vi "FPGA(test).vi"() -> ()   [LabVIEW 2019]
uses:
  <vilib>/rvi/Emulation/niFpgaGetClockAttributes.vi
  <vilib>/rvi/Emulation/niFpgaSctlEmulationGetInTimedLoop.vi
  <vilib>/rvi/Emulation/niFpgaEmulationReportErrorSimple.vi
  <vilib>/rvi/Emulation/niFpgaProcessEmulError.vi
  <vilib>/rvi/eio/common/nirviEmuTemplateMethod_errors.vi
  <vilib>/rvi/Emulation/niFpgaCriticalErrorInLSC.vi
  <vilib>/eio/EIONode/EIONode.xnode
panel:
  in  "pwm input(escon)":i32
  in  "Enable (escon)":bool
  in  "T(escon)":i32=20000
  out "Encoder(escon)":i32
  out "Encoder  (4x)":i32
  out "Encoder  (1x)":i32
  in  "encoder reset":bool
  in  "Enable":bool
  out "Encoder  (2x)":i32
  in  "stop":bool
  in  "T":i32=800000
  in  "pwm input":i32
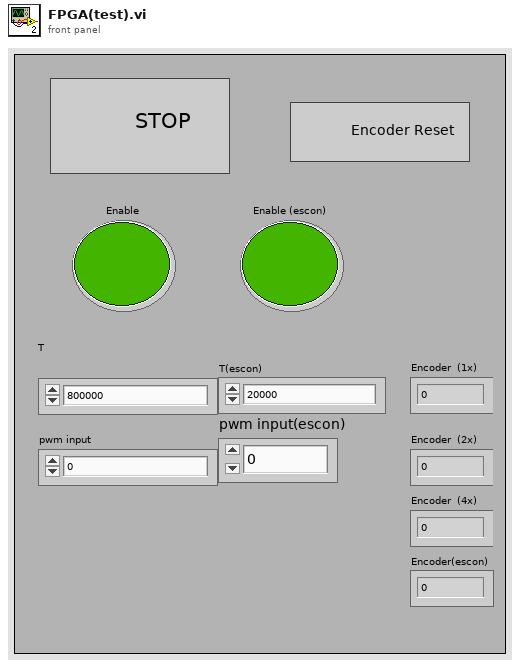
[diagram p1: front panel]
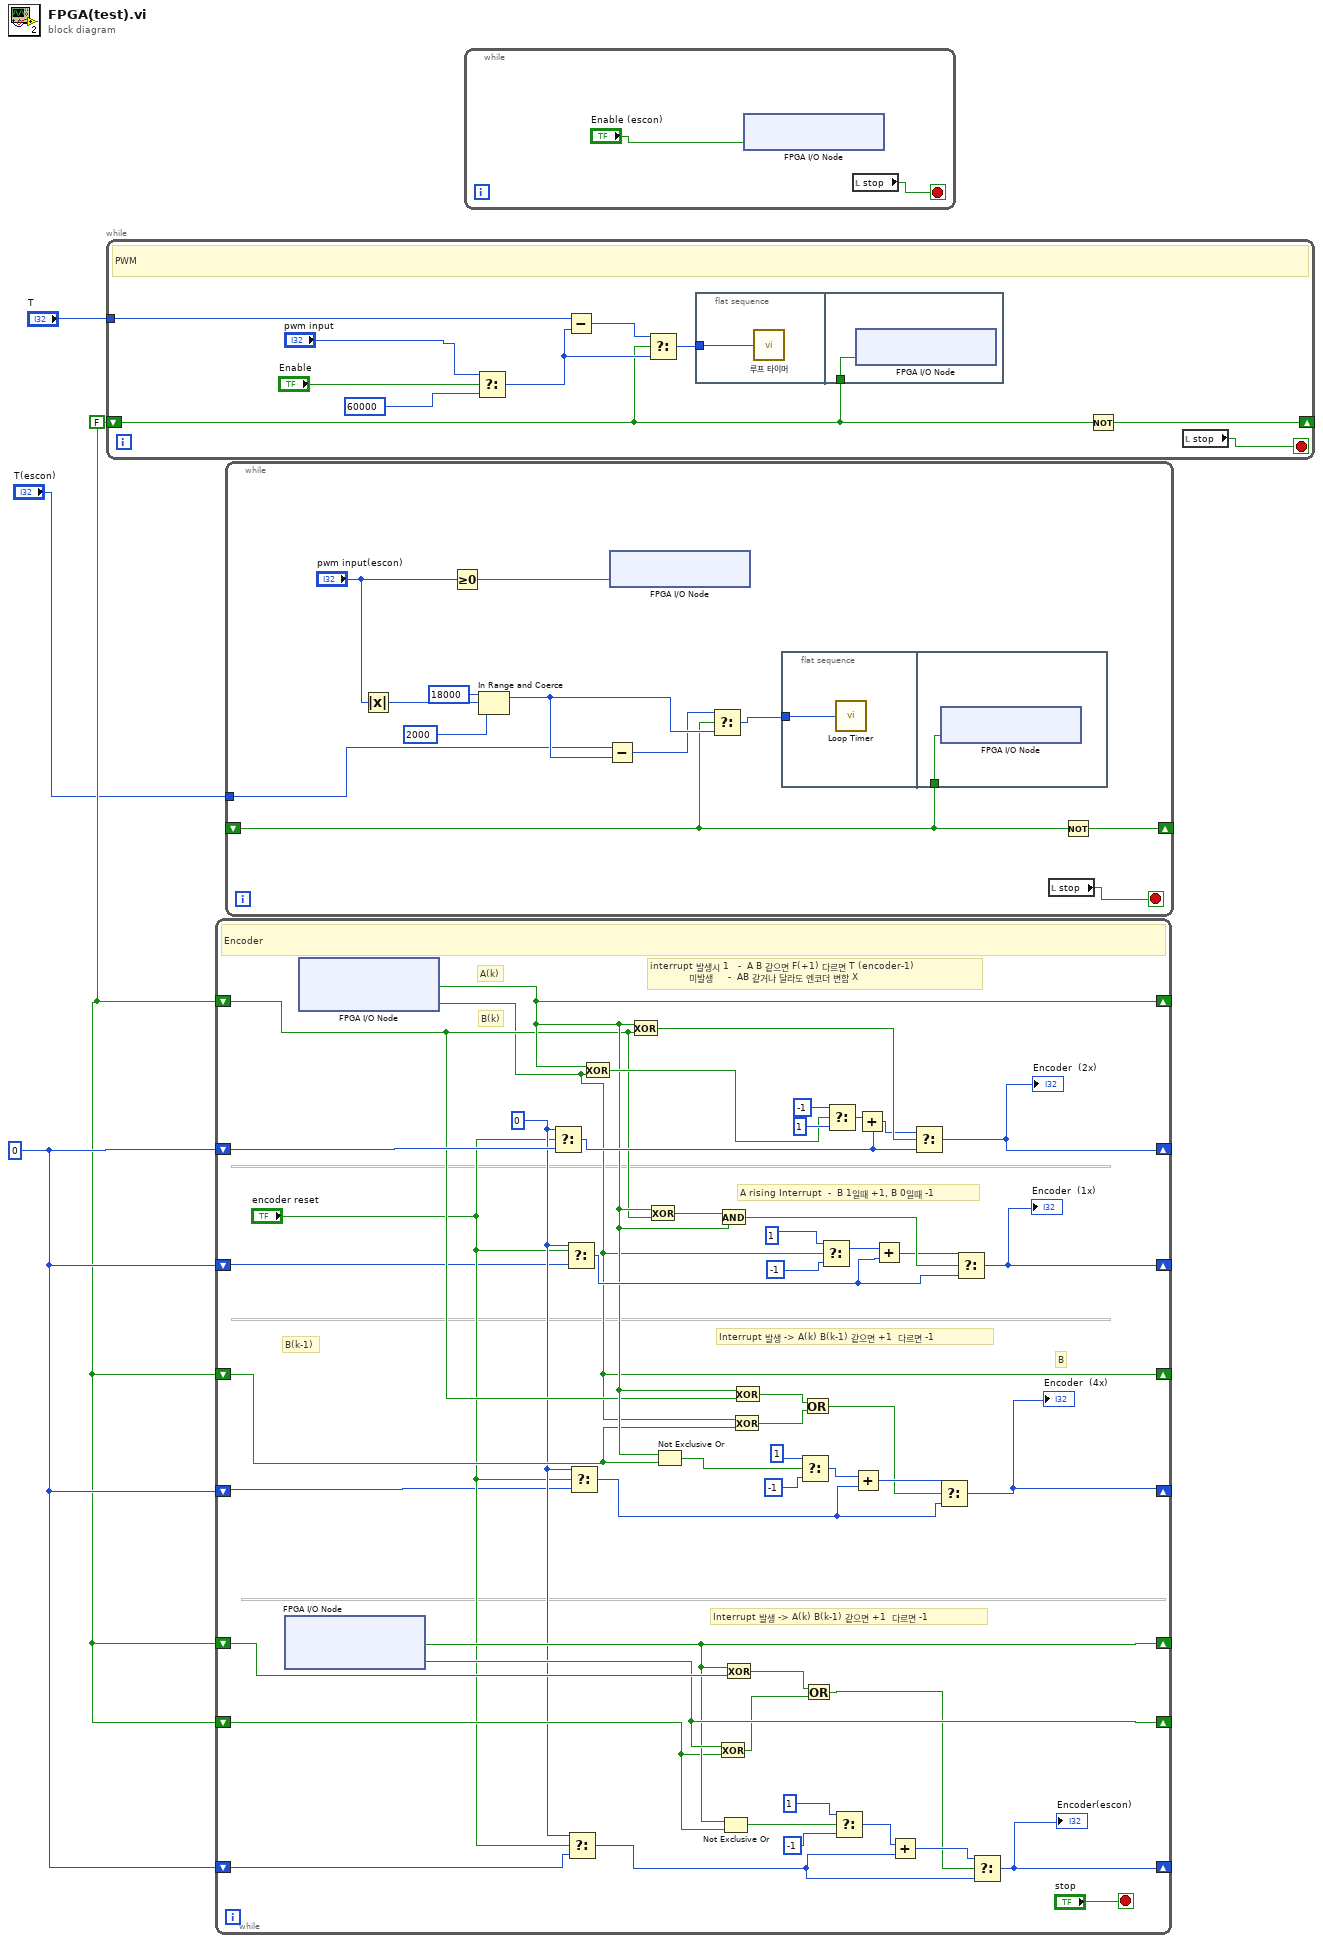
[diagram p0: block diagram]
diagram:
  w3 = 0
  w2 = FALSE
  n1 = while {
    tunnel: "T" -> [w14]
    shift-right: [w13] -> _
    shift-left: w2 -> [w6]
    stop <- w5 stop-if-true
    # "PWM"
    n2 = Select(t="pwm input", s="Enable", f=60000) -> (s? t:f=w8:i32)
    n3 = Subtract(x=w14, y=w8) -> (x-y=w12:i32)
    n4 = Select(t=w12, s=w6, f=w8) -> (s? t:f=w11:i32)
    n5 = flat-sequence {
      tunnel: w11 -> [w15]
      tunnel: w6 -> [w16]
      frame #0 {
        n6 = call "루프 타이머"("Count(Ticks)"=w15) -> ()  [unwired: 1 out]
      }
      frame #1 {
        n7 = xnode "FPGA I/O Node"("ConnectorA/DIO1"=w16) -> ()  [unwired: 1 in, 1 out]
      }
    }
    n8 = Not(x=w6) -> (.not. x?=w13:bool)
    n9 = local read "stop"() -> (w5:bool)
  }
  n10 = while {
    shift-right: [w44] -> _
    shift-left: w2 -> [w43]
    shift-right: [w39] -> _
    shift-left: w3 -> [w63]
    shift-right: [w42] -> _
    shift-left: w2 -> [w41]
    shift-right: [w33] -> _
    shift-left: w2 -> [w37]
    shift-right: [w35] -> _
    shift-left: w2 -> [w32]
    shift-right: [w25] -> _
    shift-left: w3 -> [w24]
    shift-right: [w20] -> _
    shift-left: w3 -> [w19]
    shift-right: [w18] -> _
    shift-left: w3 -> [w17]
    stop <- "stop" stop-if-true
    w22 = 0 ("t")
    # "Interrupt 발생 -> A(k) B(k-1) 같으면 +1  다르면 -1"
    # "B"
    # "B(k-1)"
    # "Interrupt 발생 -> A(k) B(k-1) 같으면 +1  다르면 -1"
    # "A rising Interrupt  -  B 1일때 +1, B 0일때 -1"
    # "B(k)"
    # "A(k)"
    # "interrupt 발생시 1   -  A B 같으면 F(+1) 다르면 T (encoder-1)\n             미발생     -  AB 같거나 달라도 엔코더 변함 X"
    # "Encoder"
    n11 = xnode "FPGA I/O Node"() -> ("ConnectorA/DIO5"=w33:bool, "ConnectorA/DIO6"=w35:bool)  [unwired: 2 in, 2 out]
    n12 = xnode "FPGA I/O Node"() -> ("ConnectorA/DIO0"=w44:bool, "ConnectorA/DIO1"=w42:bool)  [unwired: 2 in, 2 out]
    n13 = Select(t=w22, s="encoder reset", f=w63) -> (s? t:f=w62:i32)
    n14 = Select(t=w22, s="encoder reset", f=w19) -> (s? t:f=w55:i32)
    n15 = Select(t=w22, s="encoder reset", f=w24) -> (s? t:f=w23:i32)
    n16 = Select(t=w22, s="encoder reset", f=w17) -> (s? t:f=w38:i32)
    n17 = Exclusive Or(1:w42, 2:w44) -> (0:w54:bool)
    n18 = Exclusive Or(1:w43, 2:w44) -> (0:w67:bool)
    n19 = Exclusive Or(1:w43, 2:w44) -> (0:w61:bool)
    n20 = Not Exclusive Or(1:w41, 2:w44) -> (0:w50:bool)
    n21 = Exclusive Or(1:w32, 2:w35) -> (0:w34:bool)
    n22 = And(x=w61, y=w44) -> (x .and. y?=w60:bool)
    n23 = Not Exclusive Or(1:w32, 2:w33) -> (0:w31:bool)
    n24 = Exclusive Or(1:w37, 2:w33) -> (0:w36:bool)
    n25 = Exclusive Or(1:w41, 2:w42) -> (0:w46:bool)
    n26 = Exclusive Or(1:w43, 2:w44) -> (0:w47:bool)
    n27 = Select(t=i16 1, s=w50, f=i16 -1) -> (s? t:f=w49:i16)
    n28 = Or(x=w47, y=w46) -> (x .or. y?=w45:bool)
    n29 = Or(x=w36, y=w34) -> (x .or. y?=w26:bool)
    n30 = Select(t=i16 1, s=w42, f=i16 -1) -> (s? t:f=w58:i16)
    n31 = Select(t=i16 -1, s=w54, f=i16 1) -> (s? t:f=w66:i16)
    n32 = Select(t=i16 1, s=w31, f=i16 -1) -> (s? t:f=w28:i16)
    n33 = Add(x=w49, y=w38) -> (x+y=w48:i32)
    n34 = Add(x=w66, y=w62) -> (x+y=w65:i32)
    n35 = Add(x=w58, y=w55) -> (x+y=w59:i32)
    n36 = Add(x=w28, y=w23) -> (x+y=w27:i32)
    n37 = Select(t=w65, s=w67, f=w62) -> (s? t:f=w39:i32)
    "Encoder  (2x)" <- w39
    n38 = Select(t=w48, s=w45, f=w38) -> (s? t:f=w18:i32)
    "Encoder  (4x)" <- w18
    n39 = Select(t=w59, s=w60, f=w55) -> (s? t:f=w20:i32)
    "Encoder  (1x)" <- w20
    n40 = Select(t=w27, s=w26, f=w23) -> (s? t:f=w25:i32)
    "Encoder(escon)" <- w25
  }
  n41 = while {
    shift-right: [w73] -> _
    shift-left: _ -> [w72]
    tunnel: "T(escon)" -> [w71]
    stop <- w68 stop-if-true
    n42 = Absolute Value(x="pwm input(escon)") -> (abs(x)=w78:i32)
    n43 = Greater Or Equal To 0?(x="pwm input(escon)") -> (x >= 0?=w79:bool)
    n44 = In Range and Coerce(upper limit=i16 18000, x=w78, lower limit=i16 2000) -> (coerced(x)=w76:i32)  [unwired: 1 out]
    n45 = Subtract(x=w71, y=w76) -> (x-y=w75:i32)
    n46 = xnode "FPGA I/O Node"("ConnectorA/DIO3"=w79) -> ()  [unwired: 1 in, 1 out]
    n47 = Select(t=w75, s=w72, f=w76) -> (s? t:f=w74:i32)
    n48 = flat-sequence {
      tunnel: w74 -> [w80]
      tunnel: w72 -> [w81]
      frame #0 {
        n49 = call "Loop Timer"("Count(Ticks)"=w80) -> ()  [unwired: 1 out]
      }
      frame #1 {
        n50 = xnode "FPGA I/O Node"("ConnectorA/DIO2"=w81) -> ()  [unwired: 1 in, 1 out]
      }
    }
    n51 = local read "stop"() -> (w68:bool)
    n52 = Not(x=w72) -> (.not. x?=w73:bool)
  }
  n53 = while {
    stop <- w82 stop-if-true
    n54 = xnode "FPGA I/O Node"("ConnectorA/DIO5"="Enable (escon)") -> ()  [unwired: 1 in, 1 out]
    n55 = local read "stop"() -> (w82:bool)
  }
